vi "PRL Channel Selector.vi"(0 "Phasor Values In":csg[][](array[numeric]), 1 "Cut Index":i32, 2 "Get All Signals":bool, 3 "Initialize?":bool, 5 "Analog Values In":sgl[][](array[numeric]), 7 "Digital Values In":bool[][](array[boolean]), 11 "Signal Types":cluster{"Phasor":i32[], "Analog":i32[]}, 12 "Signal Names In":T1, 13 "Action":T2(ring)) -> (4 "Phasor Values Out":csg[][](array[numeric]), 6 "Analog Values Out":sgl[][](array[numeric]), 8 "Digital Values Out":bool[][](array[boolean]), 14 "Signal Names Out":T1)   [LabVIEW 2017, in "PMU Recorder Light.lvlib"]
uses:
  PMU Recorder Light.lvlib
panel:
  out "error out":errorcluster
  in  "error in (no error)":errorcluster
  in  "Digital":i32[](listbox)
  in  "Analog":i32[](listbox)
  in  "Phasor":i32[](listbox)
  # "INPUT"
  # "INTERMEDIATE"
  # "OUTPUT"
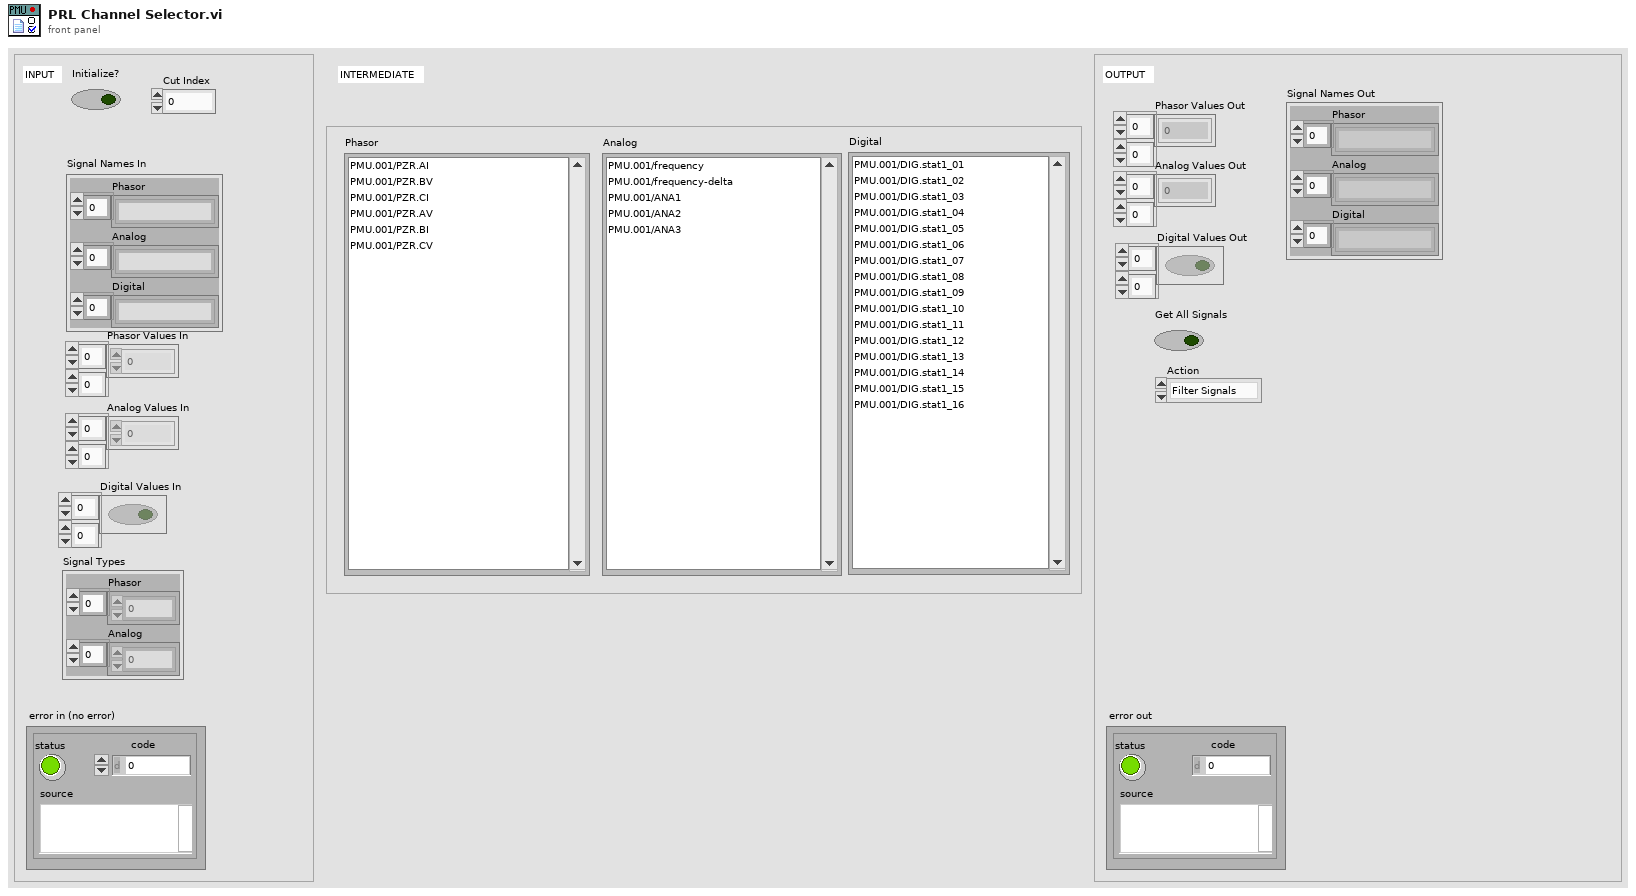
[diagram p1: front panel]
types:
  T1 = cluster{"Phasor":string[], "Analog":string[], "Digital":string[]}
  T2 = enum16{"Filter Signals", "Get All Signal Names", "Select Signals on Name", "Select Frequency Only", "Get Selected Signal Names"}
  T3 = cluster{"Item Names":string[], "Item Names":string[], "Item Names":string[]}
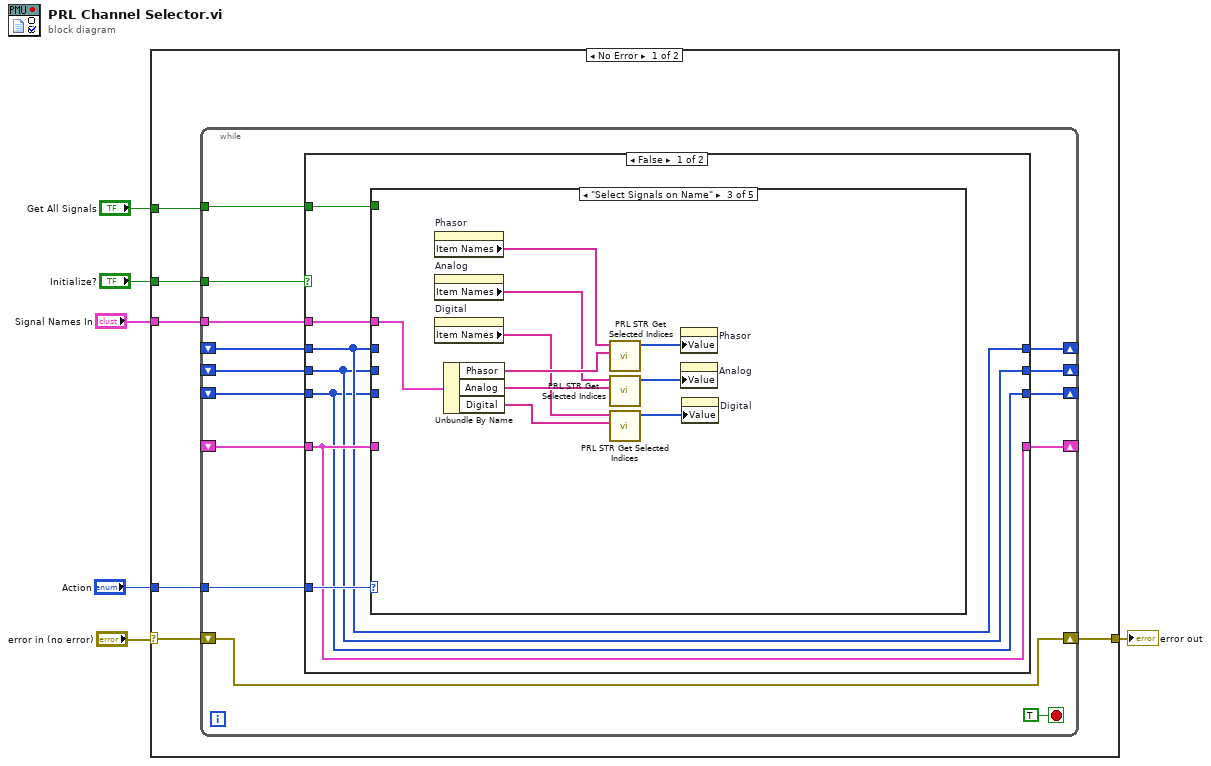
[diagram p0: block diagram]
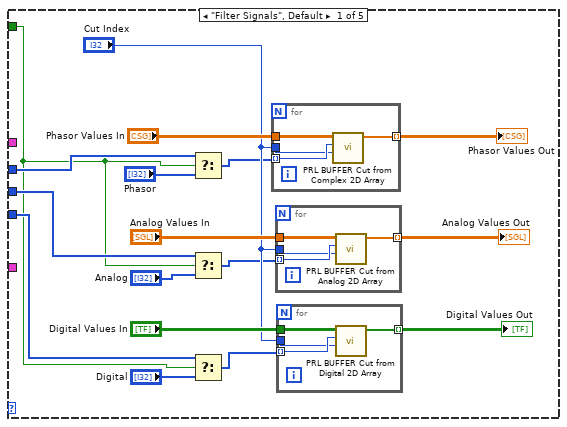
[diagram p2: hidden frame]
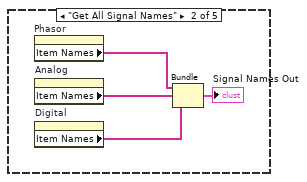
[diagram p3: hidden frame]
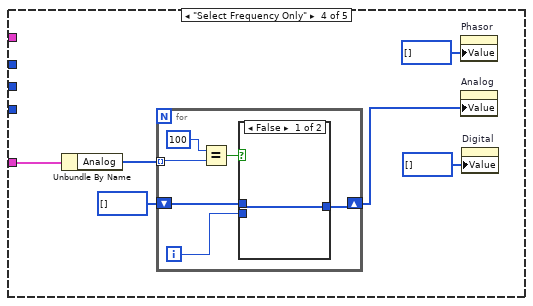
[diagram p4: hidden frame]
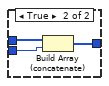
[diagram p5: hidden frame]
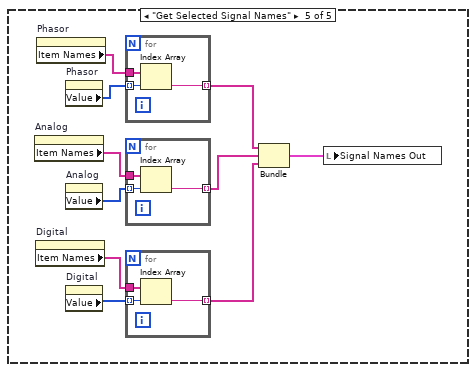
[diagram p6: hidden frame]
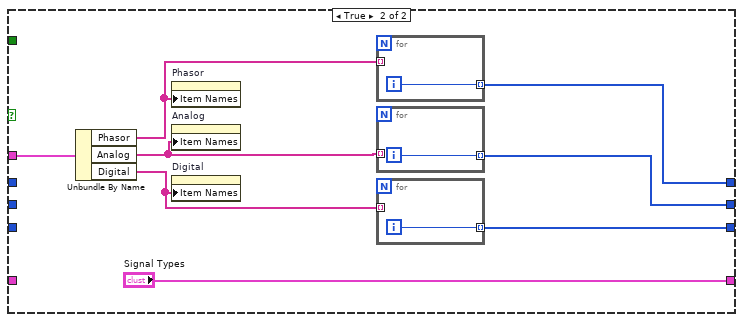
[diagram p7: hidden frame]
diagram:
  n1 = case shown="No Error" "error in (no error)" {
    selector: "error in (no error)" -> [w8 w123]
    tunnel: "Initialize?" -> [w12 _]
    tunnel: "Signal Names In" -> [w11 _]
    tunnel: "Get All Signals" -> [w10 _]
    tunnel: "Action" -> [w9 _]
    tunnel: [w7 w123] -> w1
    frame No Error {
      n2 = while {
        tunnel: w12 -> [w25]
        tunnel: w11 -> [w24]
        tunnel: w10 -> [w23]
        tunnel: w9 -> [w22]
        shift-right: [w21] -> _
        shift-left: _ -> [w20]
        shift-right: [w19] -> _
        shift-left: _ -> [w16]
        shift-right: [w18] -> _
        shift-left: _ -> [w15]
        shift-right: [w17] -> _
        shift-left: _ -> [w14]
        shift-right: [w13] -> w7
        shift-left: w8 -> [w13]
        stop <- TRUE stop-if-true
        n3 = case shown="False" w25 {
          tunnel: w24 -> [w31 w119]
          tunnel: w23 -> [w33 _]
          tunnel: w22 -> [w32 _]
          tunnel: [w30 "Signal Types"] -> w21
          tunnel: w20 -> [w30 _]
          tunnel: [w27 w114] -> w19
          tunnel: [w28 w113] -> w18
          tunnel: [w29 w112] -> w17
          tunnel: w16 -> [w27 _]
          tunnel: w15 -> [w28 _]
          tunnel: w14 -> [w29 _]
          frame False {
            n4 = case shown="\"Select Signals on Name\"" w32 {
              tunnel: w33 -> [w35 _ _ _ _]
              tunnel: w31 -> [_ _ w76 _ _]
              tunnel: w30 -> [_ _ _ w80 _]
              tunnel: w29 -> [w42 _ _ _ _]
              tunnel: w28 -> [w40 _ _ _ _]
              tunnel: w27 -> [w36 _ _ _ _]
              frame "Filter Signals", Default {
                n5 = Select(t=w42, s=w35, f="Phasor") -> (s? t:f=w38:i32[])
                n6 = Select(t=w40, s=w35, f="Analog") -> (s? t:f=w39:i32[])
                n7 = Select(t=w36, s=w35, f="Digital") -> (s? t:f=w34:i32[])
                n8 = for {
                  tunnel: "Phasor Values In" -> [w62]
                  tunnel: w38 -> [w61] mode=indexing
                  tunnel: "Cut Index" -> [w60]
                  tunnel: [w59] -> w44 mode=indexing
                  n9 = call "PRL BUFFER Cut from Complex 2D Array.vi"("Cut Index"=w60, "Signal Index"=w61, "Array In"=w62) -> ("Array Out"=w59:csg[])  [unwired: 8 in]
                }
                "Phasor Values Out" <- w44
                n10 = for {
                  tunnel: "Analog Values In" -> [w58]
                  tunnel: w39 -> [w57] mode=indexing
                  tunnel: "Cut Index" -> [w56]
                  tunnel: [w55] -> w45 mode=indexing
                  n11 = call "PRL BUFFER Cut from Analog 2D Array.vi"("Cut Index"=w56, "Signal Index"=w57, "Array In"=w58) -> ("Array Out"=w55:sgl[])  [unwired: 8 in]
                }
                "Analog Values Out" <- w45
                n12 = for {
                  tunnel: "Digital Values In" -> [w54]
                  tunnel: w34 -> [w53] mode=indexing
                  tunnel: "Cut Index" -> [w52]
                  tunnel: [w51] -> w46 mode=indexing
                  n13 = call "PRL BUFFER Cut from Digital 2D Array.vi"("Cut Index"=w52, "Signal Index"=w53, "Array In"=w54) -> ("Array Out"=w51:bool[])  [unwired: 8 in]
                }
                "Digital Values Out" <- w46
              }
              frame "Get All Signal Names" {
                n14 = property on="Phasor" class="LstBox (strict)"() -> ("Item Names"=w66:string[])  [unwired: 2 in, 2 out]
                n15 = property on="Analog" class="LstBox (strict)"() -> ("Item Names"=w65:string[])  [unwired: 2 in, 2 out]
                n16 = property on="Digital" class="LstBox (strict)"() -> ("Item Names"=w64:string[])  [unwired: 2 in, 2 out]
                n17 = Bundle("Item Names"=w66, "Item Names"=w65, "Item Names"=w64) -> (→"Signal Names Out":T3)  [unwired: 1 in]
              }
              frame "Select Signals on Name" {
                n18 = property on="Phasor" class="LstBox (strict)"() -> ("Item Names"=w75:string[])  [unwired: 2 in, 2 out]
                n19 = property on="Analog" class="LstBox (strict)"() -> ("Item Names"=w73:string[])  [unwired: 2 in, 2 out]
                n20 = property on="Digital" class="LstBox (strict)"() -> ("Item Names"=w71:string[])  [unwired: 2 in, 2 out]
                n21 = Unbundle By Name(w76) -> ("Phasor"=w74:string[], "Analog"=w72:string[], "Digital"=w70:string[])
                n22 = call "PRL STR Get Selected Indices.vi"("Selected"=w74, "All"=w75) -> ("Indices"=w69:i32[])  [unwired: 9 in]
                n23 = call "PRL STR Get Selected Indices.vi"("Selected"=w72, "All"=w73) -> ("Indices"=w68:i32[])  [unwired: 9 in]
                n24 = call "PRL STR Get Selected Indices.vi"("Selected"=w70, "All"=w71) -> ("Indices"=w67:i32[])  [unwired: 9 in]
                n25 = property on="Phasor" class="LstBox (strict)"("Value"=w69) -> ()  [unwired: 2 in, 2 out]
                n26 = property on="Analog" class="LstBox (strict)"("Value"=w68) -> ()  [unwired: 2 in, 2 out]
                n27 = property on="Digital" class="LstBox (strict)"("Value"=w67) -> ()  [unwired: 2 in, 2 out]
              }
              frame "Select Frequency Only" {
                n28 = Unbundle By Name(w80) -> ("Analog"=w79:i32[])
                n29 = for {
                  tunnel: w79 -> [w88] mode=indexing
                  shift-right: [w83] -> w77
                  shift-left: i32[] [] -> [w85]
                  i -> [w84]
                  n30 = Equal?(x=100, y=w88) -> (x = y?=w86:bool)
                  n31 = case shown="False" w86 {
                    tunnel: w85 -> [w89 w92]
                    tunnel: w84 -> [_ w91]
                    tunnel: [w89 w90] -> w83
                    frame False {
                    }
                    frame True {
                      n32 = Build Array (concatenate)(w92, w91) -> (w90:i32[])
                    }
                  }
                }
                n33 = property on="Phasor" class="LstBox (strict)"("Value"=i32[] [] ("Phasor")) -> ()  [unwired: 2 in, 2 out]
                n34 = property on="Analog" class="LstBox (strict)"("Value"=w77) -> ()  [unwired: 2 in, 2 out]
                n35 = property on="Digital" class="LstBox (strict)"("Value"=i32[] [] ("Digital")) -> ()  [unwired: 2 in, 2 out]
              }
              frame "Get Selected Signal Names" {
                n36 = property on="Analog" class="LstBox (strict)"() -> ("Item Names"=w97:string[])  [unwired: 2 in, 2 out]
                n37 = property on="Digital" class="LstBox (strict)"() -> ("Item Names"=w100:string[])  [unwired: 2 in, 2 out]
                n38 = property on="Phasor" class="LstBox (strict)"() -> ("Item Names"=w102:string[])  [unwired: 2 in, 2 out]
                n39 = property on="Phasor" class="LstBox (strict)"() -> ("Value"=w101:i32[])  [unwired: 2 in, 2 out]
                n40 = property on="Analog" class="LstBox (strict)"() -> ("Value"=w98:i32[])  [unwired: 2 in, 2 out]
                n41 = property on="Digital" class="LstBox (strict)"() -> ("Value"=w99:i32[])  [unwired: 2 in, 2 out]
                n42 = for {
                  tunnel: w102 -> [w111]
                  tunnel: w101 -> [w110] mode=indexing
                  tunnel: [w109] -> w94 mode=indexing
                  n43 = Index Array(array=w111, index=w110) -> (element=w109:string)
                }
                n44 = for {
                  tunnel: w97 -> [w108]
                  tunnel: w98 -> [w107] mode=indexing
                  tunnel: [w106] -> w96 mode=indexing
                  n45 = Index Array(array=w108, index=w107) -> (element=w106:string)
                }
                n46 = for {
                  tunnel: w100 -> [w105]
                  tunnel: w99 -> [w104] mode=indexing
                  tunnel: [w103] -> w95 mode=indexing
                  n47 = Index Array(array=w105, index=w104) -> (element=w103:string)
                }
                n48 = Bundle(w94, w96, w95) -> (w93:cluster{string[], string[], string[]})  [unwired: 1 in]
                n49 = local write "Signal Names Out"(w93) -> ()
              }
            }
          }
          frame True {
            n50 = Unbundle By Name(w119) -> ("Phasor"=w117:string[], "Analog"=w116:string[], "Digital"=w115:string[])
            n51 = property on="Phasor" class="LstBox (strict)"("Item Names"=w117) -> ()  [unwired: 2 in, 2 out]
            n52 = property on="Analog" class="LstBox (strict)"("Item Names"=w116) -> ()  [unwired: 2 in, 2 out]
            n53 = property on="Digital" class="LstBox (strict)"("Item Names"=w115) -> ()  [unwired: 2 in, 2 out]
            n54 = for {
              tunnel: w117 -> [_] mode=indexing
              tunnel: [w122] -> w112 mode=indexing
              i -> [w122]
            }
            n55 = for {
              tunnel: w116 -> [_] mode=indexing
              tunnel: [w121] -> w113 mode=indexing
              i -> [w121]
            }
            n56 = for {
              tunnel: w115 -> [_] mode=indexing
              tunnel: [w120] -> w114 mode=indexing
              i -> [w120]
            }
          }
        }
      }
    }
    frame Error {
    }
  }
  "error out" <- w1
